vi "nn allocmsg.vi"(8 "error in (no error)":errorcluster, 10 "type":i32, 11 "size":u32) -> (0 "error out":errorcluster, 3 "function return":u32)   [LabVIEW 2013, in "lvnano.lvlib"]
doc: "NN_EXPORT void *nn_allocmsg (size_t size, int type);"
uses:
  lvnano.lvlib
  get last error code.vi
  get error string from code.vi
  <vilib>/Utility/error.llb/Error Cluster From Error Code.vi
  lvnanomsg.dll
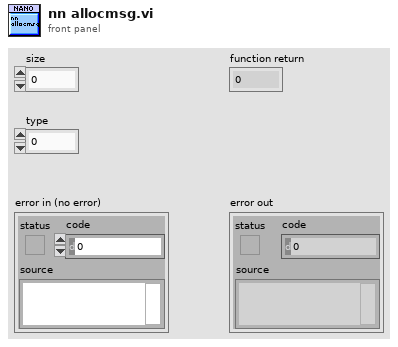
[diagram p1: front panel]
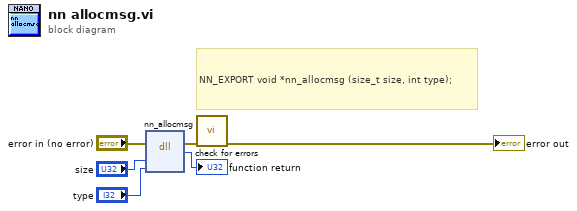
[diagram p0: block diagram]
diagram:
  # "NN_EXPORT void *nn_allocmsg (size_t size, int type);"
  n1 = dll-call lib="C:/Users/Daniel/Documents/nanomsg/lvnano/lvnanomsg.*" fn="nn_allocmsg"(error in="error in (no error)", "size"="size", "type"="type") -> (error out=w2:errorcluster, →"function return":u32)  [unwired: 4 in, 1 out]
  n2 = call "check for errors.vi"("error in"=w2) -> ("error out"=→"error out":errorcluster)  [unwired: 10 in]
